vi "SetBK120Hz.vi"(8 "error out 2":errorcluster, 11 "VISA resource name out":refnum<visa-resource-name>) -> (0 "error out":errorcluster, 3 "VISA resource name out 2":refnum<visa-resource-name>)   [LabVIEW 2021]
panel:
  out "SCPI parameter input":string[](array[string])
  out "Parameters read for device":string[](array[string])
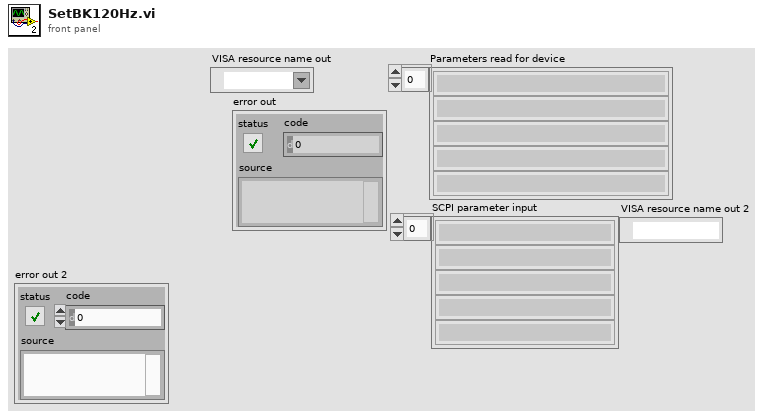
[diagram p1: front panel]
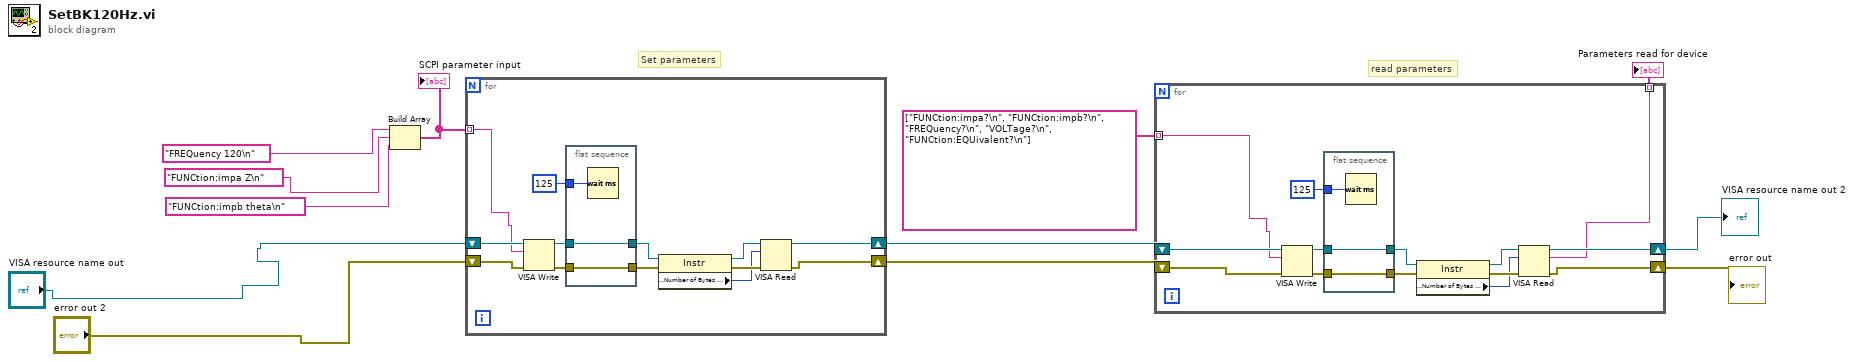
[diagram p0: block diagram]
diagram:
  # "read parameters"
  # "Set parameters"
  n1 = Build Array("FREQuency 120\n" ("element"), "FUNCtion:impa Z\n" ("element"), "FUNCtion:impb theta\n" ("element")) -> (w8:string[])
  "SCPI parameter input" <- w8
  n2 = for {
    shift-right: [w17] -> w10
    shift-left: "VISA resource name out" -> [w18]
    shift-right: [w16] -> w9
    shift-left: "error out 2" -> [w13]
    tunnel: w8 -> [w14] mode=indexing
    n3 = VISA Write(VISA resource name=w18, write buffer=w14, error in (no error)=w13) -> (VISA resource name out=w23:refnum<visa-resource-name>, error out=w25:errorcluster)  [unwired: 1 out]
    n4 = flat-sequence {
      tunnel: w25 -> [w27]
      tunnel: [w27] -> w24
      tunnel: w23 -> [w26]
      tunnel: [w26] -> w22
      tunnel: u32 125 ("delay before read (ms)") -> [w28]
      frame #0 {
        n5 = Wait (ms)(milliseconds to wait=w28) -> ()  [unwired: 1 out]
      }
    }
    n6 = property class="Instr"(reference=w22, error in=w24) -> (reference out=w21:refnum<visa-resource-name>, error out=w20:errorcluster, "Serial Settings:Number of Bytes at Serial Port"=w19:u32)
    n7 = VISA Read(VISA resource name=w21, byte count=w19, error in (no error)=w20) -> (VISA resource name out=w17:refnum<visa-resource-name>, error out=w16:errorcluster)  [unwired: 2 out]
  }
  n8 = for {
    shift-right: [w33] -> w7
    shift-left: w10 -> [w35]
    shift-right: [w32] -> w6
    shift-left: w9 -> [w34]
    tunnel: string[] ["FUNCtion:impa?\n", "FUNCtion:impb?\n", "FREQuency?\n", "VOLTage?\n", "FUNCtion:EQUivalent?\n"] -> [w30] mode=indexing
    tunnel: [w29] -> w11 mode=indexing
    n9 = VISA Write(VISA resource name=w35, write buffer=w30, error in (no error)=w34) -> (VISA resource name out=w40:refnum<visa-resource-name>, error out=w42:errorcluster)  [unwired: 1 out]
    n10 = flat-sequence {
      tunnel: w42 -> [w44]
      tunnel: [w44] -> w41
      tunnel: w40 -> [w43]
      tunnel: [w43] -> w39
      tunnel: u32 125 ("delay before read (ms)") -> [w45]
      frame #0 {
        n11 = Wait (ms)(milliseconds to wait=w45) -> ()  [unwired: 1 out]
      }
    }
    n12 = property class="Instr"(reference=w39, error in=w41) -> (reference out=w38:refnum<visa-resource-name>, error out=w37:errorcluster, "Serial Settings:Number of Bytes at Serial Port"=w36:u32)
    n13 = VISA Read(VISA resource name=w38, byte count=w36, error in (no error)=w37) -> (VISA resource name out=w33:refnum<visa-resource-name>, read buffer=w29:string, error out=w32:errorcluster)  [unwired: 1 out]
  }
  "Parameters read for device" <- w11
  "VISA resource name out 2" <- w7
  "error out" <- w6
